vi "Battle Area Rectangle.vi"() -> (3 "Viewport":T1)   [LabVIEW 2021]
uses:
  LabSDL2/Source/Libraries/LibSDL2 Wrapper/Controls/Rectangle.ctl
  Re-use Libraries/Vector 2D/Vector 2D.lvclass/Vector 2D.ctl
  Re-use Libraries/Vector 2D/Initialise.vi
  Re-use Libraries/Vector 2D/Vector 2D.lvclass
  LabSDL2/Source/Libraries/LibSDL2 Wrapper/LibSDL2.lvlib
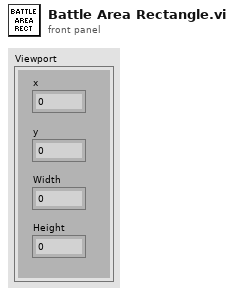
[diagram p1: front panel]
types:
  T1 = typedef "LibSDL2.lvlib/Rectangle.ctl" = cluster{"x":i32, "y":i32, "Width":i32, "Height":i32}
  T2 = typedef "Constants.ctl" = cluster{"Colours":cluster{"OK":u32, "Warning":u32, "Error":u32, "Red":u32, "Green":u32, "Blue":u32, "Yellow":u32}, "System":cluster{"Target Frames Second":dbl, "Windows Size":refnum<class "Vector 2D.lvclass">, "World Size":refnum<class "Vector 2D.lvclass">, "Battle Area Size":refnum<class "Vector 2D.lvclass">, "Sidebar Width":sgl, "SC2 Frame Rate [Seconds/Frame]":sgl, "Sidebar Player 2 Y Offset":sgl}, "Game":cluster{"Maximum Asteroids":i32, "Max Energy":i32, "Max Crew":i32, "Maximum Stars":i32}}
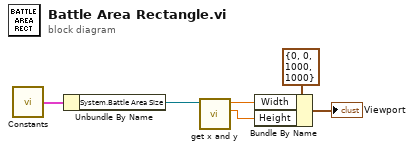
[diagram p0: block diagram]
diagram:
  n1 = call "Constants.vi"() -> ("Constants"=w6:T2)
  n2 = Unbundle By Name(w6) -> ("System.Battle Area Size"=w3:refnum<class "Vector 2D.lvclass">)
  n3 = call "get x and y.vi"("Vector 2D in"=w3) -> ("y"=w1:sgl, "x"=w2:sgl)  [unwired: 9 in]
  n4 = Bundle By Name(cluster=T1 {"x"=0, "y"=0, "Width"=1000, "Height"=1000} ("Rectangle"), "Width"=w2, "Height"=w1) -> (→"Viewport":T1)
